vi "Error Checking.vi"(8 "error in (no error)":errorcluster, 11 "VISA resource name":refnum<visa-resource-name>) -> (0 "error out":errorcluster, 2 "Connection Error":bool, 3 "VISA resource name":refnum<visa-resource-name>)   [LabVIEW 2018]
uses:
  <vilib>/Utility/error.llb/DialogType.ctl
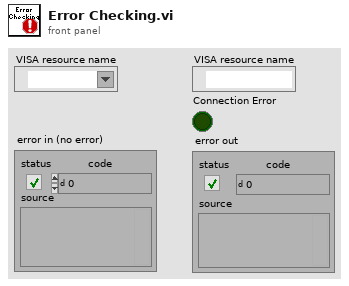
[diagram p1: front panel]
types:
  T1 = typedef "DialogType.ctl" = u16
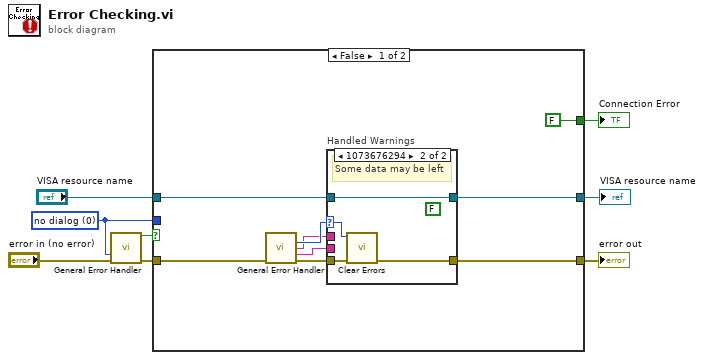
[diagram p0: block diagram]
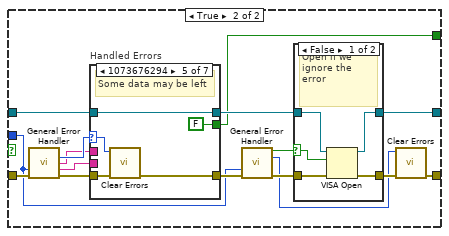
[diagram p3: hidden frame]
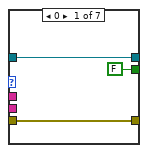
[diagram p5: hidden frame]
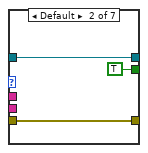
[diagram p6: hidden frame]
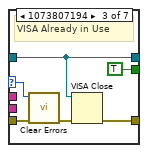
[diagram p7: hidden frame]
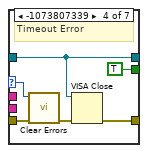
[diagram p8: hidden frame]
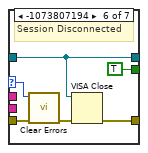
[diagram p9: hidden frame]
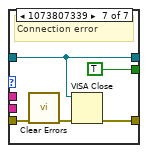
[diagram p10: hidden frame]
diagram:
  w2 = T1 0 items=["no dialog", "OK message", "continue or stop message", "OK message + warnings", "continue/stop + warnings"] ("type of dialog (OK msg:1)")
  n1 = call <vilib>:"General Error Handler.vi"("type of dialog (OK msg:1)"=w2, "error in (no error)"="error in (no error)") -> ("error?"=w8:bool, "error out"=w7:errorcluster)  [unwired: 9 in, 3 out]
  n2 = case shown="False" w8 {
    tunnel: [w9 w38] -> w6
    tunnel: w7 -> [w10 w39]
    tunnel: "VISA resource name" -> [w12 w37]
    tunnel: [w11 w31] -> w3
    tunnel: w2 -> [_ w29]
    tunnel: [FALSE w24] -> w1
    frame False {
      n3 = call <vilib>:"General Error Handler.vi"("error in (no error)"=w10) -> ("code out"=w15:i32, "source out"=w14:string, "message"=w13:string, "error out"=w16:errorcluster)  [unwired: 10 in, 1 out]
      n4 = case "Handled Warnings" shown="1073676294" w15 {
        selector: w15 -> [_ w20]
        tunnel: w16 -> [w19 w21]
        tunnel: [w19 w23] -> w9
        tunnel: w14 -> [_ _]
        tunnel: w13 -> [_ _]
        tunnel: w12 -> [w18 w22]
        tunnel: [w18 w22] -> w11
        frame Default {
        }
        frame 1073676294 {
          (unwired) FALSE
          # "Some data may be left"
          n5 = call <vilib>:"Clear Errors.vi"("error in (no error)"=w21, "specific error code to clear (0: all)"=w20) -> ("error out"=w23:errorcluster)  [unwired: 4 in, 1 out]
        }
      }
    }
    frame True {
      n6 = call <vilib>:"General Error Handler.vi"("type of dialog (OK msg:1)"=w29, "error in (no error)"=w39) -> ("code out"=w27:i32, "source out"=w26:string, "message"=w25:string, "error out"=w36:errorcluster)  [unwired: 9 in, 1 out]
      n7 = case "Handled Errors" shown="1073676294" w27 {
        selector: w27 -> [_ _ w54 w60 w66 w71 _]
        tunnel: w36 -> [w49 w52 w56 w62 w67 w73 w79]
        tunnel: [w49 w52 w58 w64 w69 w75 w77] -> w35
        tunnel: w26 -> [_ _ _ _ _ _ _]
        tunnel: w25 -> [_ _ _ _ _ _ _]
        tunnel: w37 -> [w48 w51 w57 w63 w68 w74 w78]
        tunnel: [w48 w51 w57 w63 w68 w74 w78] -> w30
        tunnel: [FALSE TRUE TRUE TRUE FALSE TRUE TRUE] -> w24
        frame 0 {
        }
        frame Default {
        }
        frame 1073807194 {
          # "VISA Already in Use"
          n8 = call <vilib>:"Clear Errors.vi"("error in (no error)"=w56, "specific error code to clear (0: all)"=w54) -> ("error out"=w55:errorcluster)  [unwired: 4 in, 1 out]
          n9 = VISA Close(VISA resource name=w57, error in (no error)=w55) -> (error out=w58:errorcluster)
        }
        frame -1073807339 {
          # "Timeout Error"
          n10 = call <vilib>:"Clear Errors.vi"("error in (no error)"=w62, "specific error code to clear (0: all)"=w60) -> ("error out"=w61:errorcluster)  [unwired: 4 in, 1 out]
          n11 = VISA Close(VISA resource name=w63, error in (no error)=w61) -> (error out=w64:errorcluster)
        }
        frame 1073676294 {
          # "Some data may be left"
          n12 = call <vilib>:"Clear Errors.vi"("error in (no error)"=w67, "specific error code to clear (0: all)"=w66) -> ("error out"=w69:errorcluster)  [unwired: 4 in, 1 out]
        }
        frame -1073807194 {
          # "Session Disconnected"
          n13 = call <vilib>:"Clear Errors.vi"("error in (no error)"=w73, "specific error code to clear (0: all)"=w71) -> ("error out"=w72:errorcluster)  [unwired: 4 in, 1 out]
          n14 = VISA Close(VISA resource name=w74, error in (no error)=w72) -> (error out=w75:errorcluster)
        }
        frame 1073807339 {
          # "Connection error"
          n15 = call <vilib>:"Clear Errors.vi"("error in (no error)"=w79) -> ("error out"=w80:errorcluster)  [unwired: 5 in, 1 out]
          n16 = VISA Close(VISA resource name=w78, error in (no error)=w80) -> (error out=w77:errorcluster)
        }
      }
      n17 = call <vilib>:"General Error Handler.vi"("type of dialog (OK msg:1)"=w29, "error in (no error)"=w35) -> ("error?"=w34:bool, "code out"=w28:i32, "error out"=w33:errorcluster)  [unwired: 9 in, 2 out]
      n18 = case shown="False" w34 {
        selector: w34 -> [w44 _]
        tunnel: [w41 w46] -> w32
        tunnel: w33 -> [w40 w46]
        tunnel: w30 -> [w43 w45]
        tunnel: [w42 w45] -> w31
        frame False {
          # "Open if we ignore the error"
          n19 = VISA Open(duplicate session (F)=w44, error in (no error)=w40, VISA resource name=w43) -> (VISA resource name=w42:refnum<visa-resource-name>, error out=w41:errorcluster)  [unwired: 2 in]
        }
        frame True {
          # "Leave it closed if we don't ignore"
        }
      }
      n20 = call <vilib>:"Clear Errors.vi"("error in (no error)"=w32, "specific error code to clear (0: all)"=w28) -> ("error out"=w38:errorcluster)  [unwired: 4 in, 1 out]
    }
  }
  "error out" <- w6
  "VISA resource name" <- w3
  "Connection Error" <- w1
